vi "Overlay adjust (line).vi"(0 "Image in":T2, 1 "Enable overlay?":bool, 2 "Measurement Name":string, 3 "Configured coordinates":cluster{"X":sgl, "Y":sgl}[](array[cluster]), 5 "Mouse release point":cluster{"X":sgl, "Y":sgl}, 7 "Line width":i32, 9 "Points array":cluster{"X":sgl, "Y":sgl}[](array[cluster]), 11 "error in (no error)":errorcluster, 12 "Color":u32(colorbox)=4349695, 13 "Inspection mode":bool, 14 "Overlay coordinates":cluster{"X":sgl, "Y":sgl}[](array[cluster])) -> (4 "Image Out":T2, 6 "Transformed line":T1, 8 "Overlay Coordinates":cluster{"X":sgl, "Y":sgl}[](array[cluster]), 10 "Mid point":cluster{"X":sgl, "Y":sgl}, 15 "error out":errorcluster)   [LabVIEW 2019]
uses:
  <vilib>/vision/Image Controls.llb/IMAQ Image.ctl
  <vilib>/vision/NI_Vision_Development_Module.lvlib
panel:
  out "Distance":dbl format="%.2f"
  out "Intersection Point":cluster{"X":sgl, "Y":sgl} {"Y" format="%.2f"; "X" format="%.2f"}
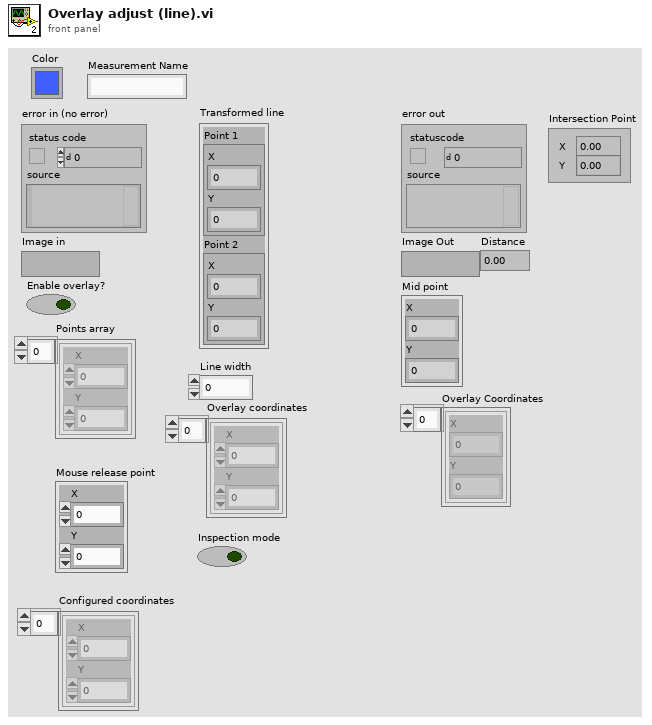
[diagram p1: front panel]
types:
  T1 = cluster{"Point 1":cluster{"X":sgl, "Y":sgl}, "Point 2":cluster{"X":sgl, "Y":sgl}}
  T2 = typedef "IMAQ Image.ctl" = refnum<image>
  T3 = typedef "IMAQ Line" = cluster{"Start X":i32, "Start Y":i32, "End X":i32, "End Y":i32}
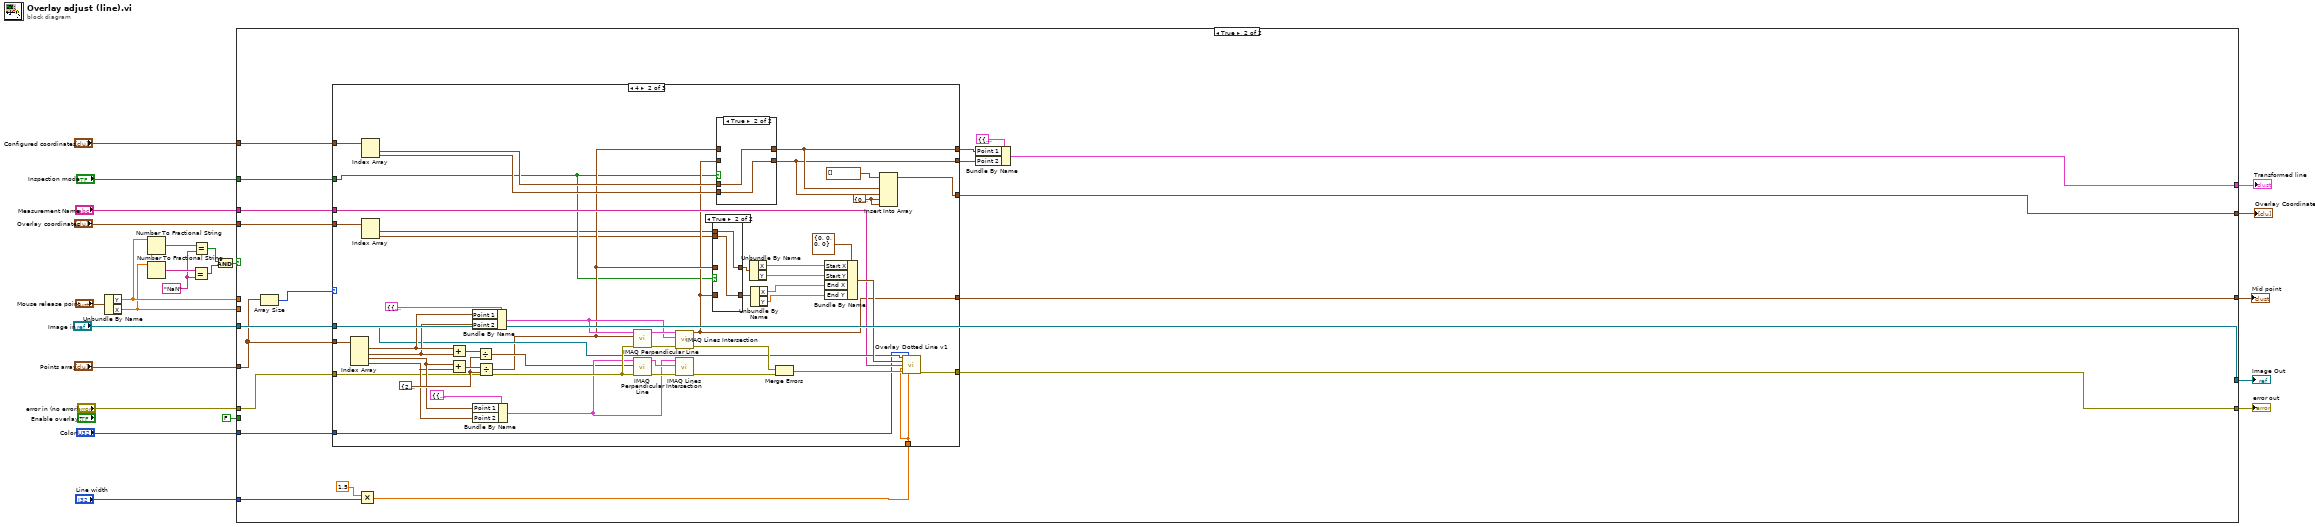
[diagram p0: block diagram]
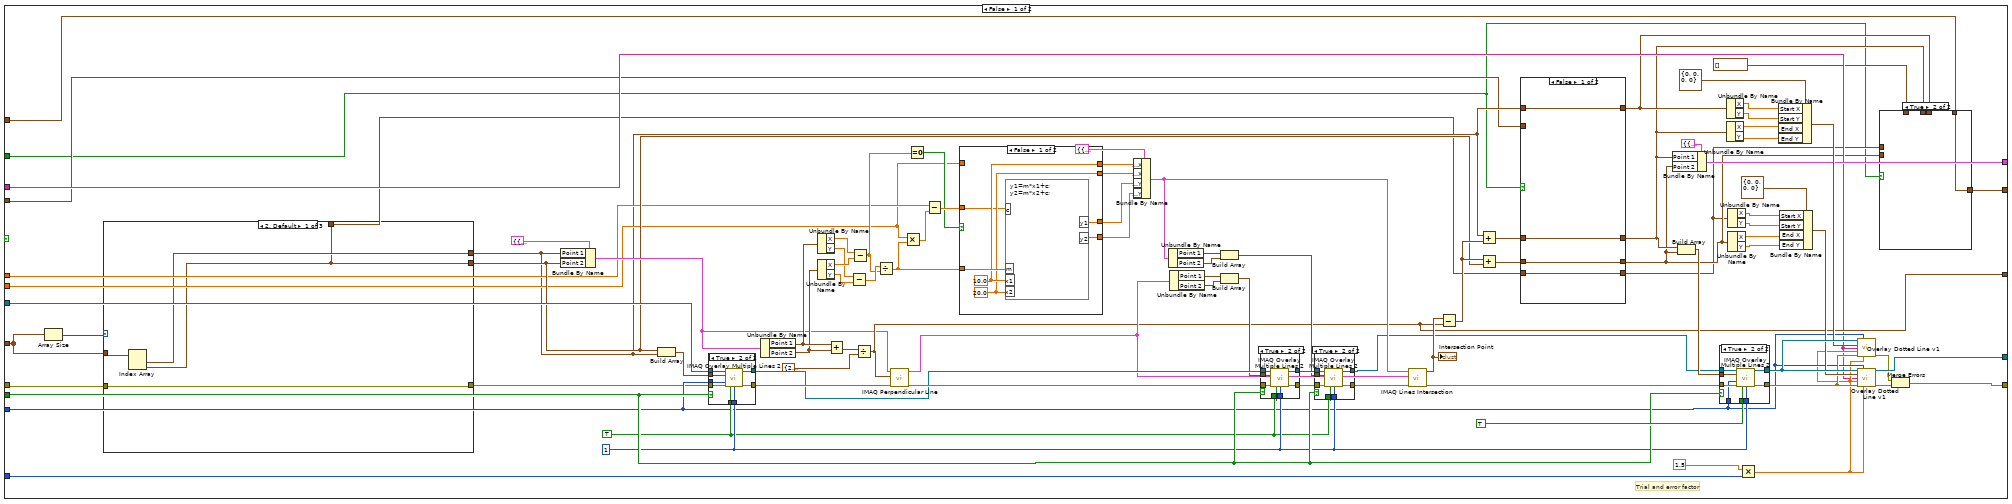
[diagram p2: hidden frame]
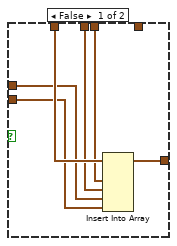
[diagram p3: hidden frame]
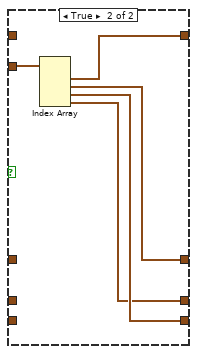
[diagram p4: hidden frame]
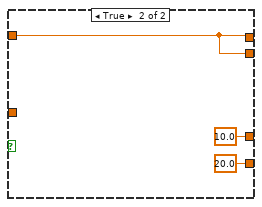
[diagram p5: hidden frame]
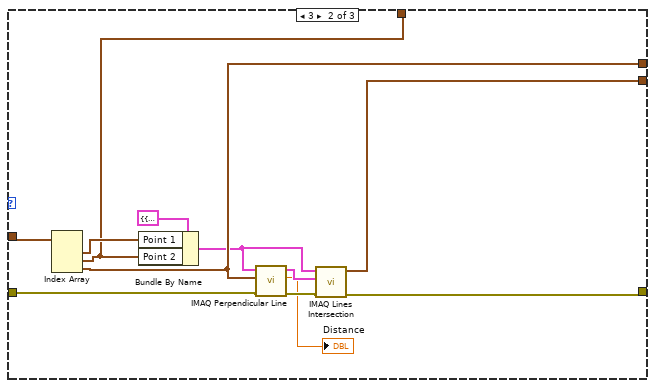
[diagram p6: hidden frame]
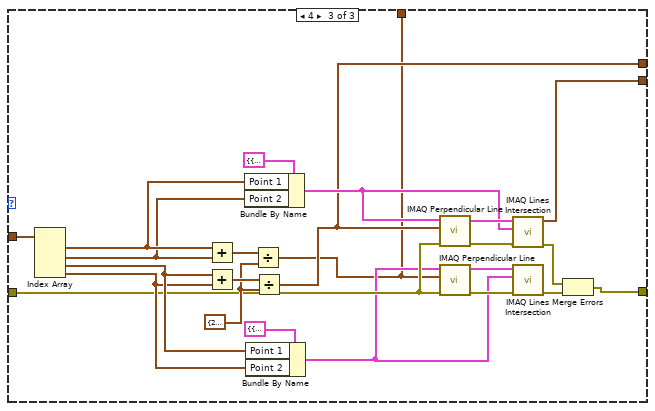
[diagram p7: hidden frame]
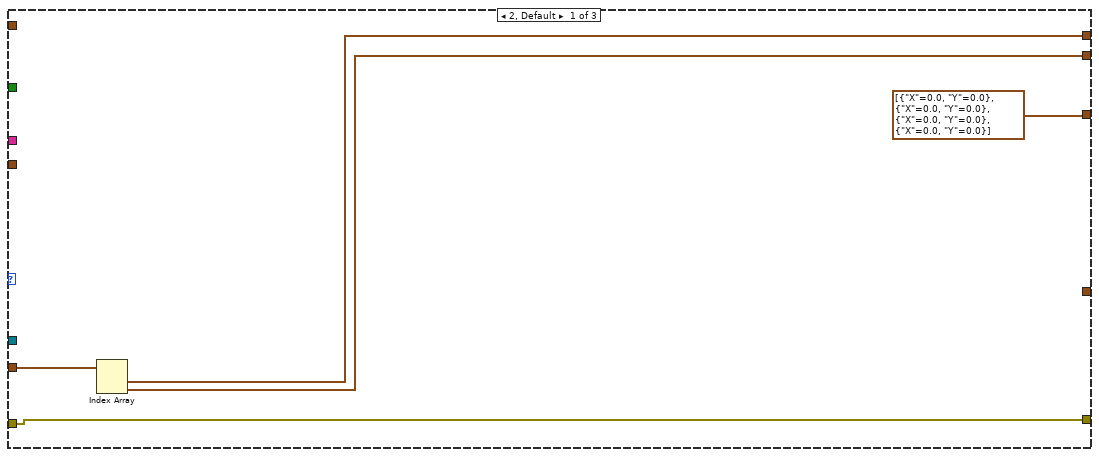
[diagram p12: hidden frame]
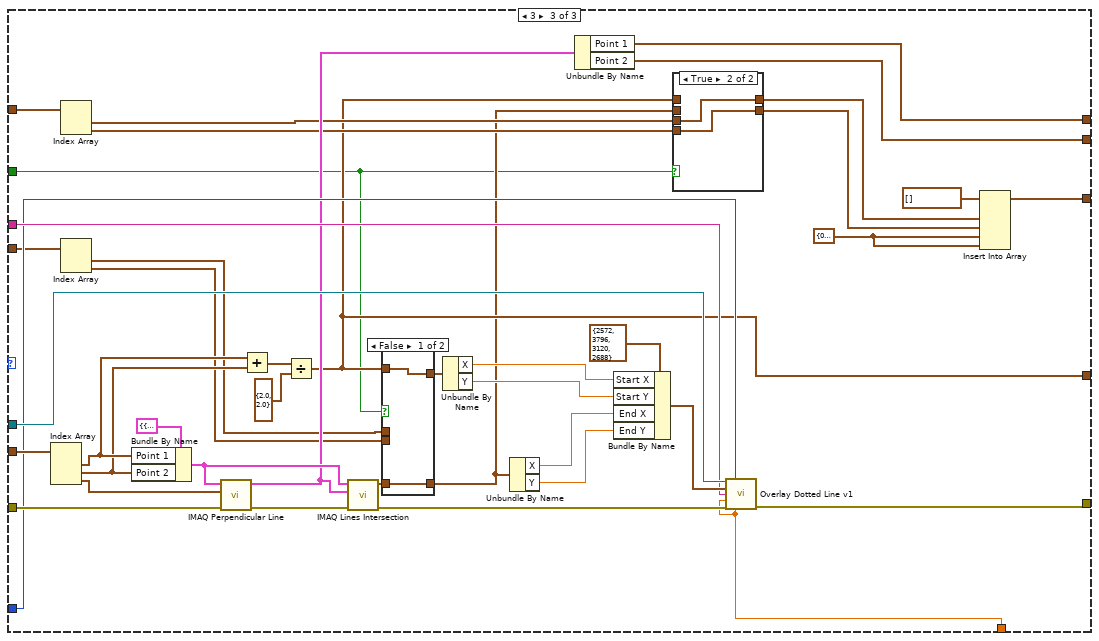
[diagram p15: hidden frame]
diagram:
  w12 = "NaN" ("y")
  n1 = Unbundle By Name("Mouse release point") -> ("Y"=w16:sgl, "X"=w15:sgl)
  n2 = Number To Fractional String(number=w16) -> (F-format string=w14:string)  [unwired: 3 in]
  n3 = Number To Fractional String(number=w15) -> (F-format string=w13:string)  [unwired: 3 in]
  n4 = Equal?(x=w13, y=w12) -> (x = y?=w11:bool)
  n5 = Equal?(x=w14, y=w12) -> (x = y?=w10:bool)
  n6 = And(x=w10, y=w11) -> (x .and. y?=w9:bool)
  n7 = case shown="True" w9 {
    tunnel: "Color" -> [w54 w223]
    tunnel: "error in (no error)" -> [w48 w237]
    tunnel: "Points array" -> [w44 w226]
    tunnel: "Image in" -> [w95 w236]
    tunnel: [w92 w236] -> w20
    tunnel: [w77 w235] -> w19
    tunnel: [w74 w227] -> w18
    tunnel: FALSE ("Enable overlay?") -> [w65 _]
    tunnel: w16 -> [w40 _]
    tunnel: w15 -> [w38 _]
    tunnel: [w53 w228] -> w8
    tunnel: "Line width" -> [w52 w234]
    tunnel: "Measurement Name" -> [w49 w232]
    tunnel: [w36 w222] -> w4
    tunnel: "Overlay coordinates" -> [w27 w220]
    tunnel: "Inspection mode" -> [w26 w221]
    tunnel: "Configured coordinates" -> [w25 w219]
    frame False {
      w64 = u32 1 ("Width")
      w63 = TRUE ("Maintain Width?")
      # "Trial and error factor"
      n8 = Array Size(array=w44) -> (size(s)=w43:i32)
      n9 = case shown="2, Default" w43 {
        tunnel: w48 -> [w144 w154 w166]
        tunnel: [w144 w152 w165] -> w47
        tunnel: w44 -> [w145 w157 w164]
        tunnel: [w142 w149 w160] -> w42
        tunnel: [w143 w155 w159] -> w35
        tunnel: [w142 w147 w158] -> w29
        frame 2, Default {
          n10 = Index Array(array=w145) -> (element #1=w143:cluster{"X":sgl, "Y":sgl}, element #2=w142:cluster{"X":sgl, "Y":sgl})  [unwired: 2 in]
        }
        frame 3 {
          n11 = Index Array(array=w157) -> (element #1=w148:cluster{"X":sgl, "Y":sgl}, element #2=w147:cluster{"X":sgl, "Y":sgl}, element #3=w155:cluster{"X":sgl, "Y":sgl})  [unwired: 3 in]
          n12 = Bundle By Name(cluster=T1 {"Point 1"={"X"=0.0, "Y"=0.0}, "Point 2"={"X"=0.0, "Y"=0.0}} ("Line"), "Point 1"=w148, "Point 2"=w147) -> (w150:T1)
          n13 = call "IMAQ Perpendicular Line"("error in (no error)"=w154, "Point"=w155, "Line"=w150) -> ("error out"=w153:errorcluster, "Distance"=→"Distance":dbl, "Perpendicular Line"=w151:T1)  [unwired: 6 in]
          n14 = call "IMAQ Lines Intersection"("error in (no error)"=w153, "Line 2"=w151, "Line 1"=w150) -> ("error out"=w152:errorcluster, "Intersection Point"=w149:cluster{"X":sgl, "Y":sgl})  [unwired: 6 in, 1 out]
        }
        frame 4 {
          w178 = cluster{"X":sgl, "Y":sgl} {"X"=2.0, "Y"=2.0} ("y")
          n15 = Index Array(array=w164) -> (element #1=w176:cluster{"X":sgl, "Y":sgl}, element #2=w175:cluster{"X":sgl, "Y":sgl}, element #3=w173:cluster{"X":sgl, "Y":sgl}, element #4=w172:cluster{"X":sgl, "Y":sgl})  [unwired: 4 in]
          n16 = Add(x=w176, y=w175) -> (x+y=w180:cluster{"X":sgl, "Y":sgl})
          n17 = Add(x=w173, y=w172) -> (x+y=w179:cluster{"X":sgl, "Y":sgl})
          n18 = Bundle By Name(cluster=T1 {"Point 1"={"X"=0.0, "Y"=0.0}, "Point 2"={"X"=0.0, "Y"=0.0}} ("Line"), "Point 1"=w176, "Point 2"=w175) -> (w161:T1)
          n19 = Bundle By Name(cluster=T1 {"Point 1"={"X"=0.0, "Y"=0.0}, "Point 2"={"X"=0.0, "Y"=0.0}} ("Line"), "Point 1"=w173, "Point 2"=w172) -> (w163:T1)
          n20 = Divide(x=w180, y=w178) -> (x/y=w158:cluster{"X":sgl, "Y":sgl})
          n21 = Divide(x=w179, y=w178) -> (x/y=w159:cluster{"X":sgl, "Y":sgl})
          n22 = call "IMAQ Perpendicular Line"("error in (no error)"=w166, "Point"=w159, "Line"=w161) -> ("error out"=w171:errorcluster, "Perpendicular Line"=w167:T1)  [unwired: 6 in, 1 out]
          n23 = call "IMAQ Perpendicular Line"("error in (no error)"=w166, "Point"=w158, "Line"=w163) -> ("error out"=w169:errorcluster, "Perpendicular Line"=w162:T1)  [unwired: 6 in, 1 out]
          n24 = call "IMAQ Lines Intersection"("error in (no error)"=w171, "Line 2"=w161, "Line 1"=w167) -> ("error out"=w170:errorcluster, "Intersection Point"=w160:cluster{"X":sgl, "Y":sgl})  [unwired: 6 in, 1 out]
          n25 = call "IMAQ Lines Intersection"("error in (no error)"=w169, "Line 2"=w163, "Line 1"=w162) -> ("error out"=w168:errorcluster)  [unwired: 6 in, 2 out]
          n26 = Merge Errors(w170, w168) -> (w165:errorcluster)
        }
      }
      n27 = Bundle By Name(cluster=T1 {"Point 1"={"X"=0.0, "Y"=0.0}, "Point 2"={"X"=0.0, "Y"=0.0}} ("Line"), "Point 1"=w35, "Point 2"=w42) -> (w45:T1)
      n28 = Build Array(w42, w35) -> (w114:cluster{"X":sgl, "Y":sgl}[])
      n29 = case shown="True" w65 {
        tunnel: w63 -> [_ w218]
        tunnel: w54 -> [_ w217]
        tunnel: w114 -> [_ w216]
        tunnel: w47 -> [w210 w215]
        tunnel: w64 -> [_ w214]
        tunnel: [w210 w213] -> w113
        tunnel: w95 -> [w209 w212]
        tunnel: [w209 w211] -> w72
        frame False {
        }
        frame True {
          n30 = call "IMAQ Overlay Multiple Lines 2"("Image"=w212, "Line End Points"=w216, "Color"=w217, "error in (no error)"=w215, "Maintain Width?"=w218, "Width"=w214) -> ("Image Out"=w211:T2, "error out"=w213:errorcluster)  [unwired: 8 in]
        }
      }
      n31 = Unbundle By Name(w45) -> ("Point 1"=w112:cluster{"X":sgl, "Y":sgl}, "Point 2"=w111:cluster{"X":sgl, "Y":sgl})
      n32 = Unbundle By Name(w112) -> ("X"=w110:sgl, "Y"=w108:sgl)
      n33 = Unbundle By Name(w111) -> ("X"=w109:sgl, "Y"=w107:sgl)
      n34 = Add(x=w112, y=w111) -> (x+y=w116:cluster{"X":sgl, "Y":sgl})
      n35 = Subtract(x=w108, y=w107) -> (x-y=w106:sgl)
      n36 = Subtract(x=w110, y=w109) -> (x-y=w41:sgl)
      n37 = Divide(x=w116, y=cluster{"X":sgl, "Y":sgl} {"X"=2.0, "Y"=2.0}) -> (x/y=w53:cluster{"X":sgl, "Y":sgl})
      n38 = Divide(x=w106, y=w41) -> (x/y=w104:sgl)
      n39 = call "IMAQ Perpendicular Line"("error in (no error)"=w113, "Point"=w53, "Line"=w45) -> ("error out"=w73:errorcluster, "Perpendicular Line"=w71:T1)  [unwired: 6 in, 1 out]
      n40 = Multiply(x=w38, y=w104) -> (x*y=w105:sgl)
      n41 = Equal To 0?(x=w41) -> (x = 0?=w39:bool)
      n42 = Subtract(x=w40, y=w105) -> (x-y=w56:sgl)
      n43 = case shown="False" w39 {
        tunnel: w104 -> [w138 _]
        tunnel: [w137 w141] -> w102
        tunnel: [w136 w141] -> w101
        tunnel: [w135 10.0 ("y1")] -> w100
        tunnel: [w134 20.0 ("y2")] -> w99
        tunnel: w56 -> [w133 _]
        tunnel: w38 -> [_ w141]
        frame False {
          w136 = 20.0 ("input variable")
          w137 = 10.0 ("input variable")
          n44 = formula code="y1=m*x1+c;\ny2=m*x2+c;"("m"=w138, "c"=w133, "x1"=w137, "x2"=w136) -> ("y2"=w134:dbl, "y1"=w135:dbl)
        }
        frame True {
        }
      }
      n45 = Bundle By Name(cluster=T1 {"Point 1"={"X"=50.0, "Y"=50.0}, "Point 2"={"X"=150.0, "Y"=150.0}} ("Line"), "Point 1.X"=w102, "Point 2.X"=w101, "Point 1.Y"=w100, "Point 2.Y"=w99) -> (w70:T1)
      n46 = Unbundle By Name(w70) -> ("Point 1"=w69:cluster{"X":sgl, "Y":sgl}, "Point 2"=w68:cluster{"X":sgl, "Y":sgl})
      n47 = Unbundle By Name(w71) -> ("Point 1"=w67:cluster{"X":sgl, "Y":sgl}, "Point 2"=w66:cluster{"X":sgl, "Y":sgl})
      n48 = Build Array(w69, w68) -> (w60:cluster{"X":sgl, "Y":sgl}[])
      n49 = Build Array(w67, w66) -> (w59:cluster{"X":sgl, "Y":sgl}[])
      n50 = case shown="True" w65 {
        tunnel: w73 -> [w190 w198]
        tunnel: [w190 w197] -> w58
        tunnel: w72 -> [w191 w196]
        tunnel: [w191 w195] -> w62
        tunnel: w59 -> [_ w194]
        tunnel: w63 -> [_ w192]
        tunnel: w64 -> [_ w193]
        frame False {
        }
        frame True {
          n51 = call "IMAQ Overlay Multiple Lines 2"("Image"=w196, "Line End Points"=w194, "error in (no error)"=w198, "Maintain Width?"=w192, "Width"=w193) -> ("Image Out"=w195:T2, "error out"=w197:errorcluster)  [unwired: 9 in]
        }
      }
      n52 = case shown="True" w65 {
        tunnel: w58 -> [w181 w184]
        tunnel: [w181 w183] -> w57
        tunnel: w62 -> [w182 w189]
        tunnel: [w182 w188] -> w61
        tunnel: w60 -> [_ w187]
        tunnel: w63 -> [_ w185]
        tunnel: w64 -> [_ w186]
        frame False {
        }
        frame True {
          n53 = call "IMAQ Overlay Multiple Lines 2"("Image"=w189, "Line End Points"=w187, "error in (no error)"=w184, "Maintain Width?"=w185, "Width"=w186) -> ("Image Out"=w188:T2, "error out"=w183:errorcluster)  [unwired: 9 in]
        }
      }
      n54 = call "IMAQ Lines Intersection"("error in (no error)"=w57, "Line 2"=w71, "Line 1"=w70) -> ("error out"=w97:errorcluster, "Intersection Point"=w98:cluster{"X":sgl, "Y":sgl})  [unwired: 6 in, 1 out]
      "Intersection Point" <- w98
      n55 = Subtract(x=w98, y=w53) -> (x-y=w93:cluster{"X":sgl, "Y":sgl})
      n56 = Add(x=w35, y=w93) -> (x+y=w32:cluster{"X":sgl, "Y":sgl})
      n57 = Add(x=w93, y=w42) -> (x+y=w31:cluster{"X":sgl, "Y":sgl})
      n58 = case shown="False" w26 {
        tunnel: [w127 w131] -> w34
        tunnel: w35 -> [w127 _]
        tunnel: [w126 w130] -> w33
        tunnel: w32 -> [w126 _]
        tunnel: w31 -> [w125 _]
        tunnel: [w125 w128] -> w30
        tunnel: w29 -> [w124 _]
        tunnel: [w124 w129] -> w28
        tunnel: w27 -> [_ w132]
        frame False {
        }
        frame True {
          n59 = Index Array(array=w132) -> (element #1=w131:cluster{"X":sgl, "Y":sgl}, element #2=w130:cluster{"X":sgl, "Y":sgl}, element #3=w129:cluster{"X":sgl, "Y":sgl}, element #4=w128:cluster{"X":sgl, "Y":sgl})  [unwired: 4 in]
        }
      }
      n60 = Bundle By Name(cluster=T1 {"Point 1"={"X"=0.0, "Y"=0.0}, "Point 2"={"X"=0.0, "Y"=0.0}} ("Transformed line"), "Point 1"=w33, "Point 2"=w30) -> (w74:T1)
      n61 = Build Array(w33, w30) -> (w96:cluster{"X":sgl, "Y":sgl}[])
      n62 = case shown="True" w65 {
        tunnel: w97 -> [w199 w208]
        tunnel: w96 -> [_ w207]
        tunnel: w54 -> [_ w206]
        tunnel: TRUE ("Maintain Width?") -> [_ w205]
        tunnel: w64 -> [_ w204]
        tunnel: [w199 w203] -> w79
        tunnel: [w200 w202] -> w91
        tunnel: w61 -> [w200 w201]
        frame False {
        }
        frame True {
          n63 = call "IMAQ Overlay Multiple Lines 2"("Image"=w201, "Line End Points"=w207, "Color"=w206, "error in (no error)"=w208, "Maintain Width?"=w205, "Width"=w204) -> ("Image Out"=w202:T2, "error out"=w203:errorcluster)  [unwired: 8 in]
        }
      }
      n64 = Unbundle By Name(w34) -> ("X"=w83:sgl, "Y"=w82:sgl)
      n65 = Unbundle By Name(w33) -> ("X"=w89:sgl, "Y"=w88:sgl)
      n66 = Unbundle By Name(w28) -> ("X"=w85:sgl, "Y"=w84:sgl)
      n67 = Unbundle By Name(w30) -> ("X"=w87:sgl, "Y"=w86:sgl)
      n68 = Multiply(x=1.5, y=w52) -> (x*y=w51:dbl)
      n69 = Bundle By Name(cluster=T3 {"Start X"=0, "Start Y"=0, "End X"=0, "End Y"=0} ("Line"), "Start X"=w83, "Start Y"=w82, "End X"=w89, "End Y"=w88) -> (w81:T3)
      n70 = Bundle By Name(cluster=T3 {"Start X"=0, "Start Y"=0, "End X"=0, "End Y"=0} ("Line"), "Start X"=w85, "Start Y"=w84, "End X"=w87, "End Y"=w86) -> (w80:T3)
      n71 = call "Overlay Dotted Line v1.vi"("Imae in"=w91, "Color"=w54, "Line"=w81, "Measurement Name"=w49, "alternative factor"=w51, "error in (no error)"=w79, "Point Diameter (5)"=w51) -> ("error out"=w76:errorcluster)  [unwired: 7 in, 1 out]
      n72 = call "Overlay Dotted Line v1.vi"("Imae in"=w91, "Color"=w54, "Line"=w80, "Measurement Name"=w49, "alternative factor"=w51, "error in (no error)"=w79, "Point Diameter (5)"=w51) -> ("Image"=w92:T2, "error out"=w78:errorcluster)  [unwired: 7 in]
      n73 = case shown="True" w26 {
        tunnel: cluster{"X":sgl, "Y":sgl}[] [] ("Overlay Coordinates") -> [w122 _]
        tunnel: [w121 w123] -> w36
        tunnel: w34 -> [w120 _]
        tunnel: w33 -> [w119 _]
        tunnel: w30 -> [w118 _]
        tunnel: w28 -> [w117 _]
        tunnel: w25 -> [_ w123]
        frame False {
          n74 = Insert Into Array(array=w122, new element #1=w120, new element #2=w119, new element #3=w117, new element #4=w118) -> (w121:cluster{"X":sgl, "Y":sgl}[])  [unwired: 1 in]
        }
        frame True {
        }
      }
      n75 = Merge Errors(w76, w78) -> (w77:errorcluster)
    }
    frame True {
      n76 = Array Size(array=w226) -> (size(s)=w225:i32)
      n77 = Multiply(x=1.5, y=w234) -> (x*y=w231:dbl)
      n78 = case shown="4" w225 {
        tunnel: w237 -> [w241 w276 w337]
        tunnel: w236 -> [_ w267 w321]
        tunnel: [w241 w266 w328] -> w235
        tunnel: w232 -> [_ w265 w320]
        tunnel: w231 -> [_ w264 w319]
        tunnel: [w240 w257 w316] -> w229
        tunnel: [_ w248 w305] -> w228
        tunnel: w226 -> [w242 w261 w339]
        tunnel: [w239 w256 w315] -> w224
        tunnel: w223 -> [_ w260 w318]
        tunnel: [cluster{"X":sgl, "Y":sgl}[] [{"X"=0.0, "Y"=0.0}, {"X"=0.0, "Y"=0.0}, {"X"=0.0, "Y"=0.0}, {"X"=0.0, "Y"=0.0}] ("Overlay Coordinates") w258 w313] -> w222
        tunnel: w221 -> [_ w246 w302]
        tunnel: w220 -> [_ w255 w310]
        tunnel: w219 -> [_ w254 w309]
        frame 2, Default {
          n79 = Index Array(array=w242) -> (element #1=w240:cluster{"X":sgl, "Y":sgl}, element #2=w239:cluster{"X":sgl, "Y":sgl})  [unwired: 2 in]
        }
        frame 4 {
          w243 = cluster{"X":sgl, "Y":sgl} {"X"=0.0, "Y"=0.0} ("new element/subarray")
          w288 = cluster{"X":sgl, "Y":sgl} {"X"=2.0, "Y"=2.0} ("y")
          n80 = Index Array(array=w261) -> (element #1=w286:cluster{"X":sgl, "Y":sgl}, element #2=w285:cluster{"X":sgl, "Y":sgl}, element #3=w283:cluster{"X":sgl, "Y":sgl}, element #4=w282:cluster{"X":sgl, "Y":sgl})  [unwired: 4 in]
          n81 = Index Array(array=w254) -> (element #1=w253:cluster{"X":sgl, "Y":sgl}, element #2=w252:cluster{"X":sgl, "Y":sgl})  [unwired: 2 in]
          n82 = Index Array(array=w255) -> (element #1=w245:cluster{"X":sgl, "Y":sgl}, element #2=w244:cluster{"X":sgl, "Y":sgl})  [unwired: 2 in]
          n83 = Add(x=w286, y=w285) -> (x+y=w290:cluster{"X":sgl, "Y":sgl})
          n84 = Add(x=w283, y=w282) -> (x+y=w289:cluster{"X":sgl, "Y":sgl})
          n85 = Bundle By Name(cluster=T1 {"Point 1"={"X"=0.0, "Y"=0.0}, "Point 2"={"X"=0.0, "Y"=0.0}} ("Line"), "Point 1"=w286, "Point 2"=w285) -> (w262:T1)
          n86 = Bundle By Name(cluster=T1 {"Point 1"={"X"=0.0, "Y"=0.0}, "Point 2"={"X"=0.0, "Y"=0.0}} ("Line"), "Point 1"=w283, "Point 2"=w282) -> (w263:T1)
          n87 = Divide(x=w290, y=w288) -> (x/y=w250:cluster{"X":sgl, "Y":sgl})
          n88 = Divide(x=w289, y=w288) -> (x/y=w249:cluster{"X":sgl, "Y":sgl})
          n89 = call "IMAQ Perpendicular Line"("error in (no error)"=w276, "Point"=w249, "Line"=w262) -> ("error out"=w281:errorcluster, "Perpendicular Line"=w278:T1)  [unwired: 6 in, 1 out]
          n90 = call "IMAQ Perpendicular Line"("error in (no error)"=w276, "Point"=w250, "Line"=w263) -> ("error out"=w279:errorcluster, "Perpendicular Line"=w277:T1)  [unwired: 6 in, 1 out]
          n91 = call "IMAQ Lines Intersection"("error in (no error)"=w281, "Line 2"=w262, "Line 1"=w278) -> ("error out"=w280:errorcluster, "Intersection Point"=w248:cluster{"X":sgl, "Y":sgl})  [unwired: 6 in, 1 out]
          n92 = call "IMAQ Lines Intersection"("error in (no error)"=w279, "Line 2"=w277, "Line 1"=w263) -> ("error out"=w275:errorcluster)  [unwired: 6 in, 2 out]
          n93 = case shown="True" w246 {
            tunnel: [w292 w294] -> w251
            tunnel: w249 -> [w292 _]
            tunnel: w248 -> [w291 _]
            tunnel: [w291 w293] -> w247
            tunnel: w245 -> [_ w294]
            tunnel: w244 -> [_ w293]
            frame False {
            }
            frame True {
            }
          }
          n94 = case shown="True" w246 {
            tunnel: [w296 w298] -> w257
            tunnel: w249 -> [w296 _]
            tunnel: [w295 w297] -> w256
            tunnel: w248 -> [w295 _]
            tunnel: w253 -> [_ w298]
            tunnel: w252 -> [_ w297]
            frame False {
            }
            frame True {
            }
          }
          n95 = Unbundle By Name(w251) -> ("X"=w273:sgl, "Y"=w272:sgl)
          n96 = Unbundle By Name(w247) -> ("X"=w271:sgl, "Y"=w270:sgl)
          n97 = Merge Errors(w280, w275) -> (w269:errorcluster)
          n98 = Bundle By Name(cluster=T3 {"Start X"=0, "Start Y"=0, "End X"=0, "End Y"=0} ("Line"), "Start X"=w273, "Start Y"=w272, "End X"=w271, "End Y"=w270) -> (w268:T3)
          n99 = Insert Into Array(array=cluster{"X":sgl, "Y":sgl}[] [] ("Overlay Coordinates"), new element #1=w257, new element #2=w256, new element #3=w243, new element #4=w243) -> (w258:cluster{"X":sgl, "Y":sgl}[])  [unwired: 1 in]
          n100 = call "Overlay Dotted Line v1.vi"("Imae in"=w267, "Color"=w260, "Line"=w268, "Measurement Name"=w265, "alternative factor"=w264, "error in (no error)"=w269, "Point Diameter (5)"=w264) -> ("error out"=w266:errorcluster)  [unwired: 7 in, 1 out]
        }
        frame 3 {
          w299 = cluster{"X":sgl, "Y":sgl} {"X"=0.0, "Y"=0.0} ("new element/subarray")
          n101 = Index Array(array=w339) -> (element #1=w333:cluster{"X":sgl, "Y":sgl}, element #2=w332:cluster{"X":sgl, "Y":sgl}, element #3=w336:cluster{"X":sgl, "Y":sgl})  [unwired: 3 in]
          n102 = Index Array(array=w309) -> (element #1=w308:cluster{"X":sgl, "Y":sgl}, element #2=w307:cluster{"X":sgl, "Y":sgl})  [unwired: 2 in]
          n103 = Index Array(array=w310) -> (element #1=w301:cluster{"X":sgl, "Y":sgl}, element #2=w300:cluster{"X":sgl, "Y":sgl})  [unwired: 2 in]
          n104 = Bundle By Name(cluster=T1 {"Point 1"={"X"=0.0, "Y"=0.0}, "Point 2"={"X"=0.0, "Y"=0.0}} ("Line"), "Point 1"=w333, "Point 2"=w332) -> (w334:T1)
          n105 = call "IMAQ Perpendicular Line"("error in (no error)"=w337, "Point"=w336, "Line"=w334) -> ("error out"=w335:errorcluster, "Perpendicular Line"=w317:T1)  [unwired: 6 in, 1 out]
          n106 = Add(x=w333, y=w332) -> (x+y=w331:cluster{"X":sgl, "Y":sgl})
          n107 = Divide(x=w331, y=cluster{"X":sgl, "Y":sgl} {"X"=2.0, "Y"=2.0}) -> (x/y=w305:cluster{"X":sgl, "Y":sgl})
          n108 = call "IMAQ Lines Intersection"("error in (no error)"=w335, "Line 2"=w317, "Line 1"=w334) -> ("error out"=w329:errorcluster, "Intersection Point"=w303:cluster{"X":sgl, "Y":sgl})  [unwired: 6 in, 1 out]
          n109 = case shown="False" w302 {
            tunnel: [w341 w343] -> w306
            tunnel: w305 -> [w341 _]
            tunnel: [w340 w342] -> w304
            tunnel: w303 -> [w340 _]
            tunnel: w301 -> [_ w343]
            tunnel: w300 -> [_ w342]
            frame False {
            }
            frame True {
            }
          }
          n110 = Unbundle By Name(w306) -> ("X"=w326:sgl, "Y"=w325:sgl)
          n111 = Unbundle By Name(w304) -> ("X"=w324:sgl, "Y"=w323:sgl)
          n112 = Unbundle By Name(w317) -> ("Point 1"=w316:cluster{"X":sgl, "Y":sgl}, "Point 2"=w315:cluster{"X":sgl, "Y":sgl})
          n113 = Bundle By Name(cluster=T3 {"Start X"=2572, "Start Y"=3796, "End X"=3120, "End Y"=2688} ("Line"), "Start X"=w326, "Start Y"=w325, "End X"=w324, "End Y"=w323) -> (w322:T3)
          n114 = case shown="True" w302 {
            tunnel: w305 -> [w345 _]
            tunnel: w304 -> [w344 _]
            tunnel: [w345 w347] -> w312
            tunnel: [w344 w346] -> w311
            tunnel: w308 -> [_ w347]
            tunnel: w307 -> [_ w346]
            frame False {
            }
            frame True {
            }
          }
          n115 = call "Overlay Dotted Line v1.vi"("Imae in"=w321, "Color"=w318, "Line"=w322, "Measurement Name"=w320, "alternative factor"=w319, "error in (no error)"=w329, "Point Diameter (5)"=w319) -> ("error out"=w328:errorcluster)  [unwired: 7 in, 1 out]
          n116 = Insert Into Array(array=cluster{"X":sgl, "Y":sgl}[] [] ("Overlay Coordinates"), new element #1=w312, new element #2=w311, new element #3=w299, new element #4=w299) -> (w313:cluster{"X":sgl, "Y":sgl}[])  [unwired: 1 in]
        }
      }
      n117 = Bundle By Name(cluster=T1 {"Point 1"={"X"=0.0, "Y"=0.0}, "Point 2"={"X"=0.0, "Y"=0.0}} ("Transformed line"), "Point 1"=w229, "Point 2"=w224) -> (w227:T1)
    }
  }
  "error out" <- w19
  "Image Out" <- w20
  "Transformed line" <- w18
  "Mid point" <- w8
  "Overlay Coordinates" <- w4
